vi "getHelp.vi"(8 "error in (no error)":errorcluster, 10 "Functions":T1="Binarizer", 11 "Scikit-learn in":refnum<class "Scikit-learn.lvclass">) -> (0 "error out":errorcluster, 2 "String":string, 3 "Scikit-learn out":refnum<class "Scikit-learn.lvclass">)   [LabVIEW 2020, in "Scikit-learn.lvclass"]
uses:
  Scikit-learn.lvclass
  Controls/ctl_Functions.ctl
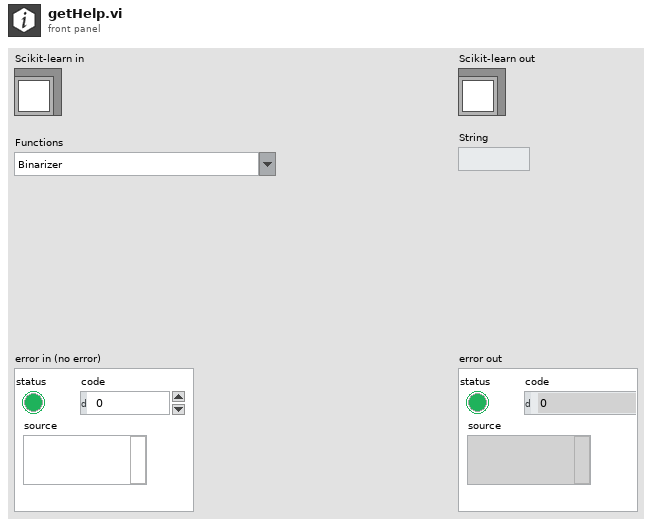
[diagram p1: front panel]
types:
  T1 = typedef "ctl_Functions.ctl" = string
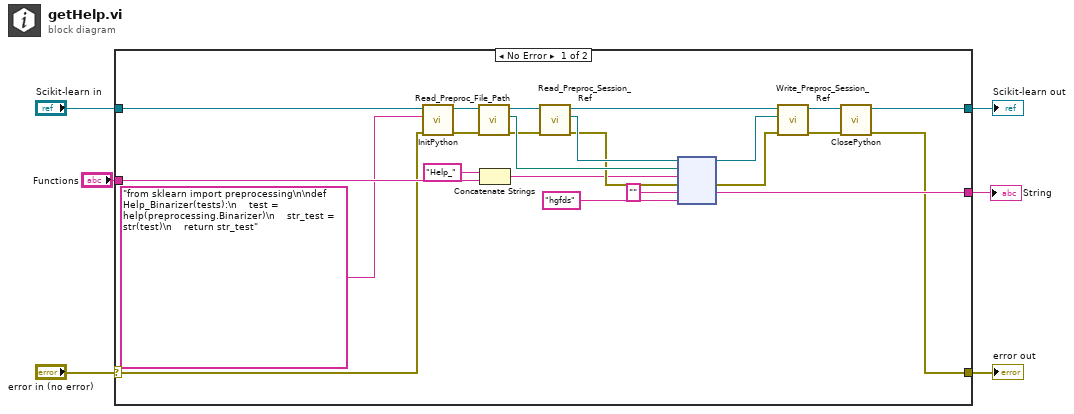
[diagram p0: block diagram]
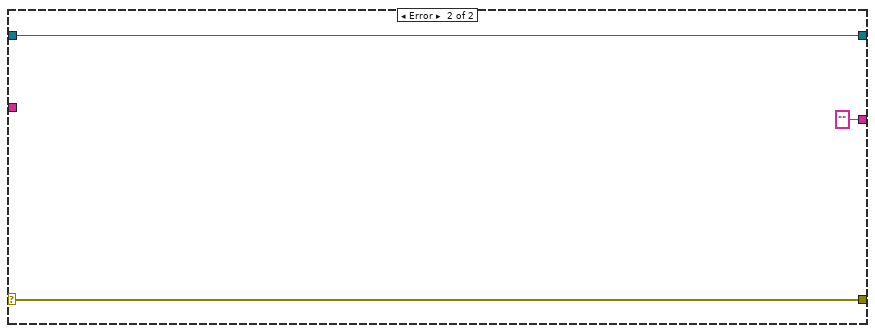
[diagram p2: hidden frame]
diagram:
  n1 = case shown="No Error" "error in (no error)" {
    selector: "error in (no error)" -> [w8 w32]
    tunnel: [w9 w32] -> w5
    tunnel: [w10 w31] -> w3
    tunnel: "Scikit-learn in" -> [w16 w31]
    tunnel: [w20 ""] -> w1
    tunnel: "Functions" -> [w17 _]
    frame No Error {
      n2 = call-dynamic "InitPython.vi"("error in (no error)"=w8, "Python Instruction"="from sklearn import preprocessing\n\ndef Help_Binarizer(tests):\n    test = help(preprocessing.Binarizer)\n    str_test = str(test)\n    return str_test", "Scikit-learn en entrée"=w16) -> ("error out"=w14:errorcluster, "Scikit-learn en sortie"=w15:refnum<class "Scikit-learn.lvclass">)  [unwired: 7 in]
      n3 = call-dynamic "Read_Preproc_File_Path.vi"("error in (no error)"=w14, "Python in"=w15) -> ("error out"=w24:errorcluster, "File_Path"=w27:path, "Python out"=w29:refnum<class "Scikit-learn.lvclass">)  [unwired: 7 in]
      n4 = Concatenate Strings("Help_", w17) -> (w18:string)
      n5 = call-dynamic "Read_Preproc_Session_Ref.vi"("error in (no error)"=w24, "Python in"=w29) -> ("error out"=w25:errorcluster, "Session_ref"=w26:refnum<k35>, "Python out"=w28:refnum<class "Scikit-learn.lvclass">)  [unwired: 7 in]
      n6 = node(w26, w27, w18, w25, "", "hgfds") -> (w21:refnum<k35>, w23:errorcluster, w20:string)  [unwired: 1 in, 2 out]
      n7 = call-dynamic "Write_Preproc_Session_Ref.vi"("error in (no error)"=w23, "Session_ref"=w21, "Python in"=w28) -> ("error out"=w11:errorcluster, "Python out"=w12:refnum<class "Scikit-learn.lvclass">)  [unwired: 7 in]
      n8 = call-dynamic "ClosePython.vi"("error in (no error)"=w11, "Scikit-learn en entrée"=w12) -> ("error out"=w9:errorcluster, "Scikit-learn en sortie"=w10:refnum<class "Scikit-learn.lvclass">)  [unwired: 8 in]
    }
    frame Error {
    }
  }
  "error out" <- w5
  "Scikit-learn out" <- w3
  "String" <- w1
